vi "50kwh battery decode.vi"(11 "data out":string) -> (0 "F-format string":string[](array[string]), 3 "output array":u32[](array[numeric]))   [LabVIEW 2021]
panel:
  in  "Tab Control":T1(tab)
  out "Main Subsea Battery - 148 V DC, 50 kWh":T2 {"Battery \nPower" scale=0.0..50.0; "SOC" scale=0.0..100.0; "Temp" scale=0.0..50.0; "Bat \nCurrent" scale=0.0..250.0; "Bat\n voltage" scale=0.0..180.0}
  out "Battery Modules":string[][](table)
  out "Battery 1 fault":bool
  out "Battery 2 fault":bool
  out "Battery 3 fault":bool
  out "Battery 4 fault":bool
  out "Battery 5 fault":bool
  out "Battery 1 warn":bool
  out "Battery 2 warn":bool
  out "Battery 3 warn":bool
  out "Battery 4 warn":bool
  out "Battery 5 warn":bool
  out "Battery stat 1":bool
  out "Battery stat 2":bool
  out "Battery stat 3":bool
  out "Battery stat 4":bool
  out "Battery stat 5":bool
  out "Battery Pack 5":T3 {"Power" scale=0.0..10.0; "SOC" scale=0.0..100.0; "Temp" scale=0.0..60.0; "Bat Current" scale=0.0..50.0; "Bat Voltage" scale=0.0..200.0}
  out "Battery Pack 4":T3 {"Power" scale=0.0..10.0; "SOC" scale=0.0..100.0; "Temp" scale=0.0..60.0; "Bat Current" scale=0.0..50.0; "Bat Voltage" scale=0.0..200.0}
  out "Battery Pack 3":T3 {"Power" scale=0.0..10.0; "SOC" scale=0.0..100.0; "Temp" scale=0.0..60.0; "Bat Current" scale=0.0..50.0; "Bat Voltage" scale=0.0..200.0}
  out "Battery Pack 2":T3 {"Power" scale=0.0..10.0; "SOC" scale=0.0..100.0; "Temp" scale=0.0..60.0; "Bat Current" scale=0.0..50.0; "Bat Voltage" scale=0.0..200.0}
  out "Battery Pack 1":T3 {"Power" scale=0.0..10.0; "SOC" scale=0.0..100.0; "Temp" scale=0.0..60.0; "Bat Current" scale=0.0..50.0; "Bat Voltage" scale=0.0..200.0}
  out "length":i32
  out "max .Volt cell":dbl
  out "max. cell ID":dbl
  out "max .C.B.ID":dbl
  out "Min .Volt cell":dbl
  out "Min.Cell.ID":dbl
  out "min.C.B.ID":dbl
  out "x = y?":bool
  out "input":i32
  # "National Institute of Ocean Technology\nMatsya 6000 - Battery System"
  # "kW"
  # "°C"
  # "%"
  # "V"
  # "A"
  # "Bat 4"
  # "Bat 2"
  # "Bat 3"
  # "Bat 1"
  # "Bat 5"
  # "Status"
  # "Warnings"
  # "Faults"
  # "V"
  # "A"
  # "°C"
  # "%"
  # "kW"
  # "V"
  # "A"
  # "°C"
  # "%"
  # "kW"
  # "V"
  # "A"
  # "°C"
  # "%"
  # "kW"
  # "V"
  # "A"
  # "°C"
  # "%"
  # "kW"
  # "V"
  # "A"
  # "°C"
  # "%"
  # "kW"
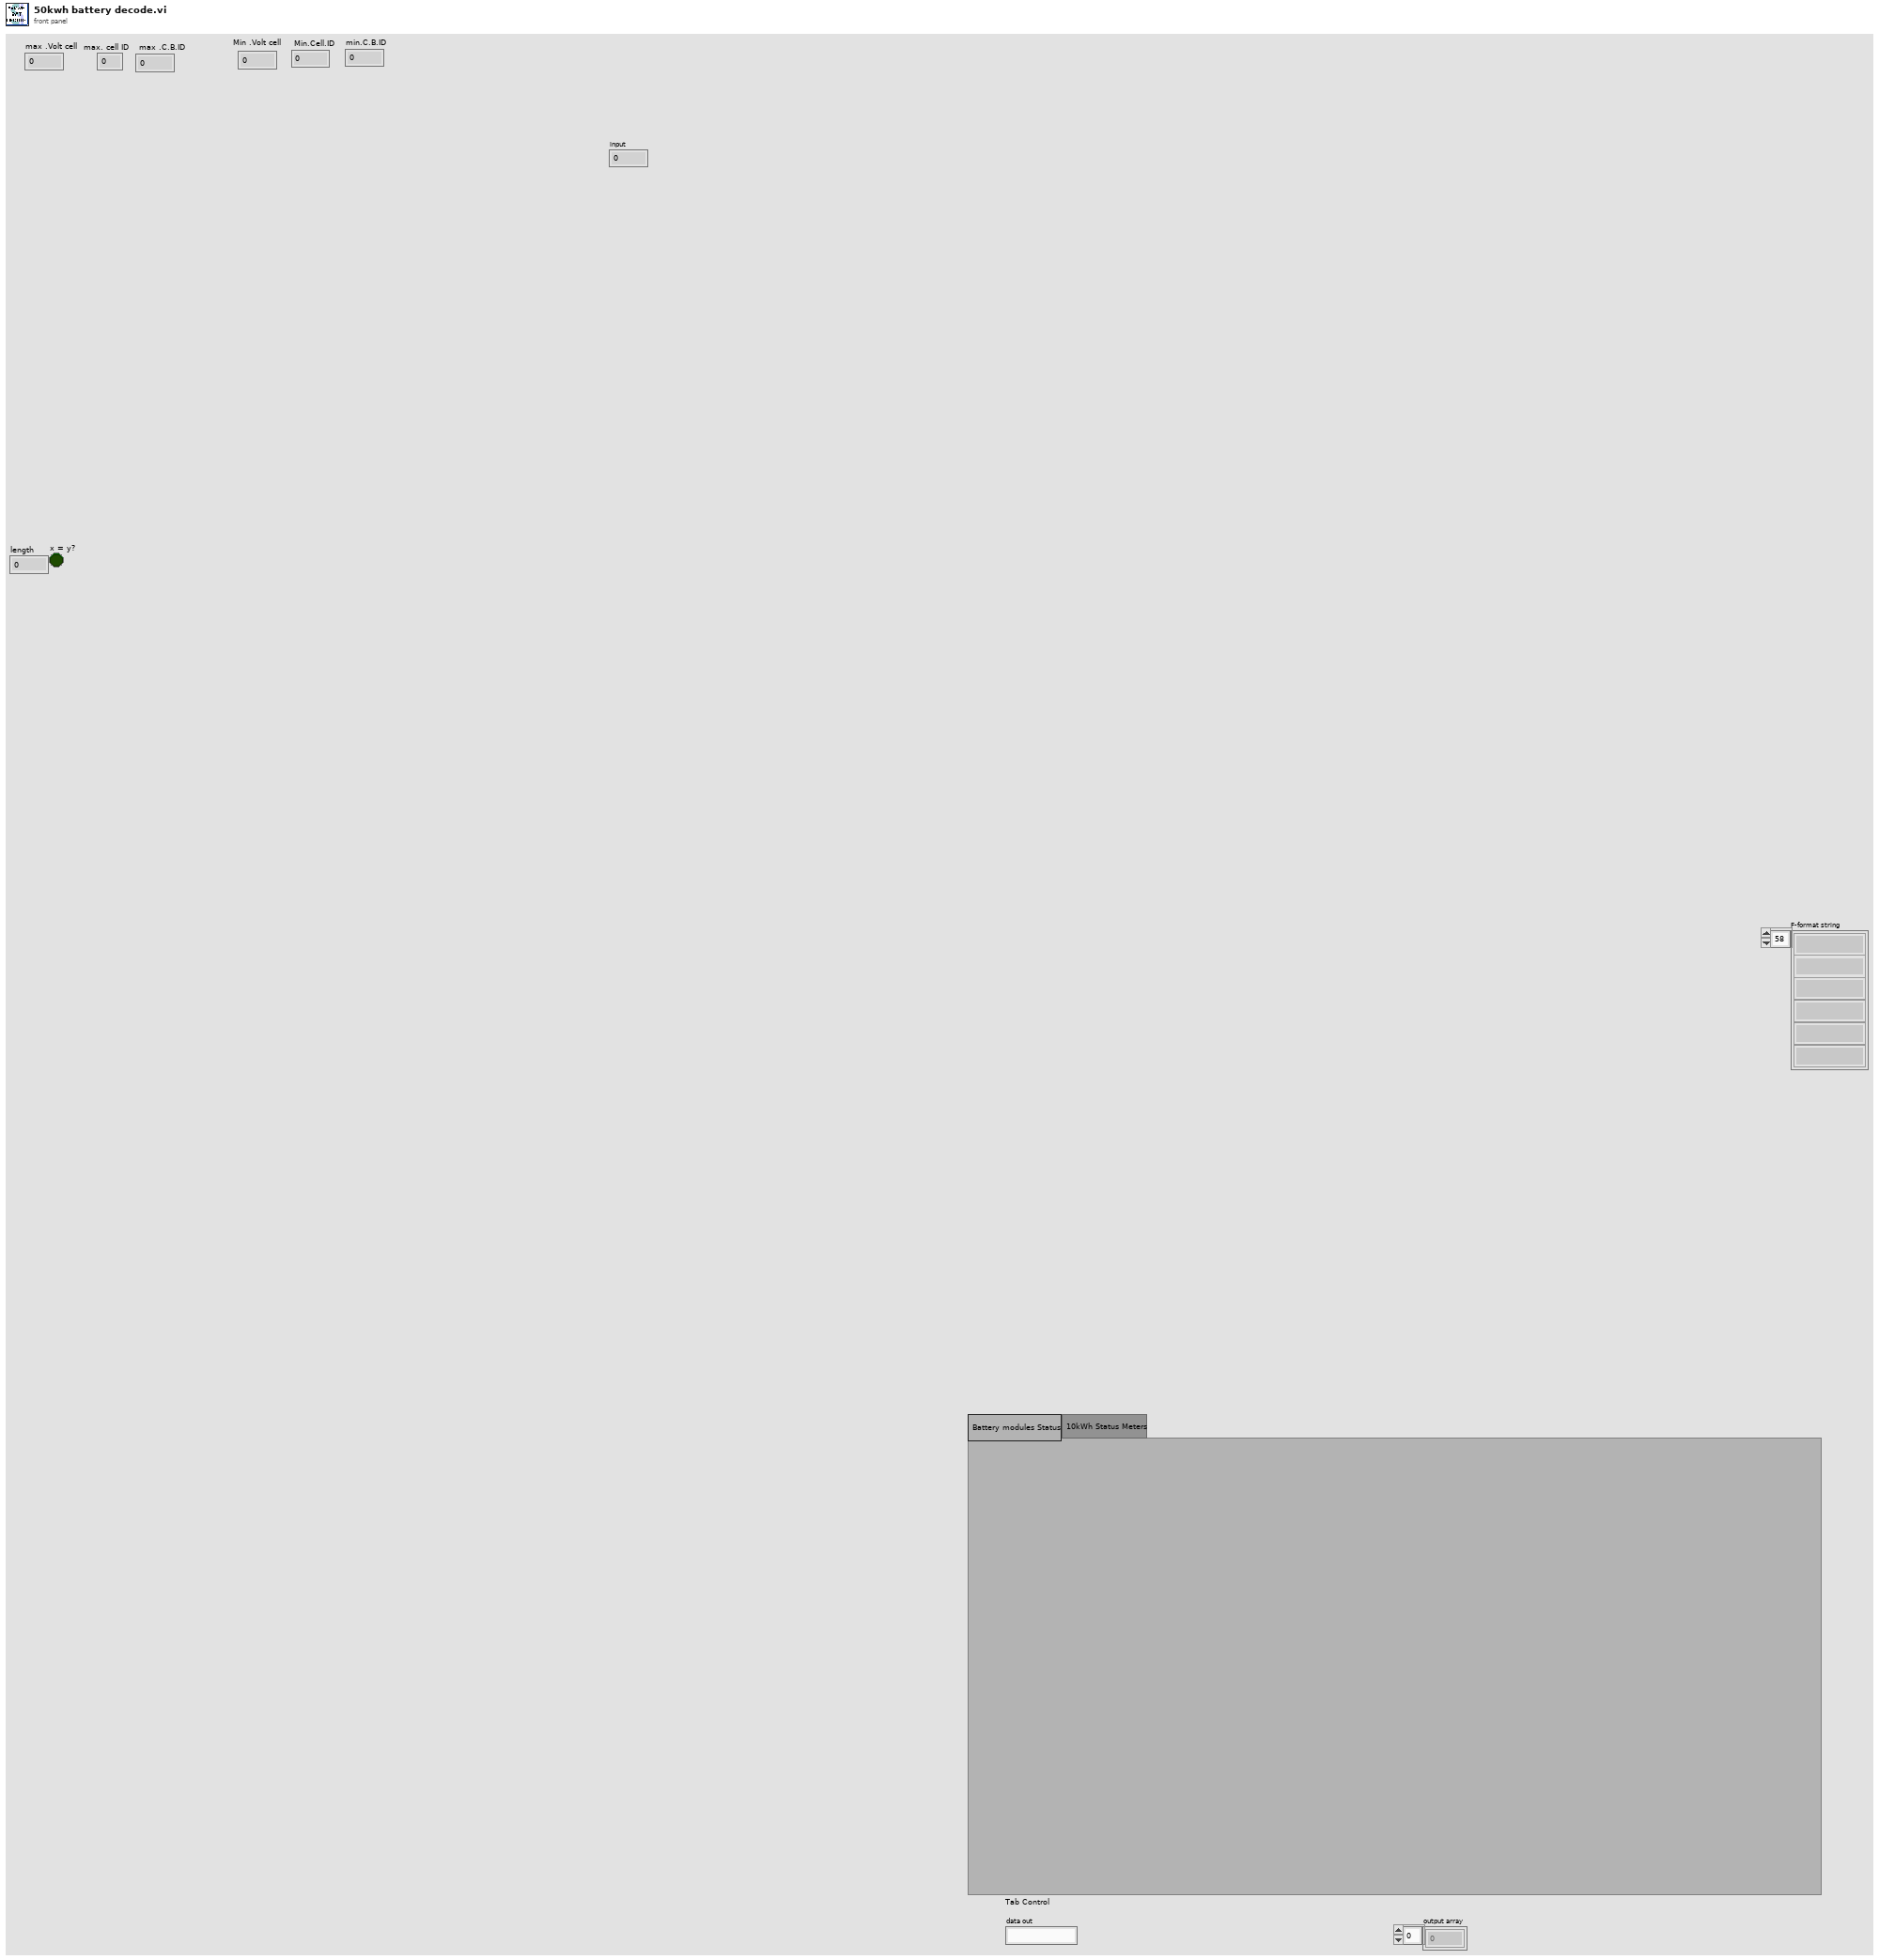
[diagram p1: front panel]
types:
  T1 = enum32{"Battery modules Status", "10kWh Status Meters"}
  T2 = cluster{"Bat\n voltage":u8, "Bat \nCurrent":u8, "Temp":u8, "SOC":u8, "Battery \nPower":sgl}
  T3 = cluster{"Bat Voltage":u16, "Bat Current":u16, "Temp":u8, "SOC":u8, "Power":sgl}
  T4 = cluster{"Numeric":u8, "Numeric":u8, "Numeric":u8, "Numeric":u8, dbl}
  T5 = cluster{u16, u16, "Numeric":u8, "Numeric":u8, dbl}
  T6 = cluster{"Numeric":u8, "Numeric":u8, "Numeric":u8, "Numeric":u8, sgl}
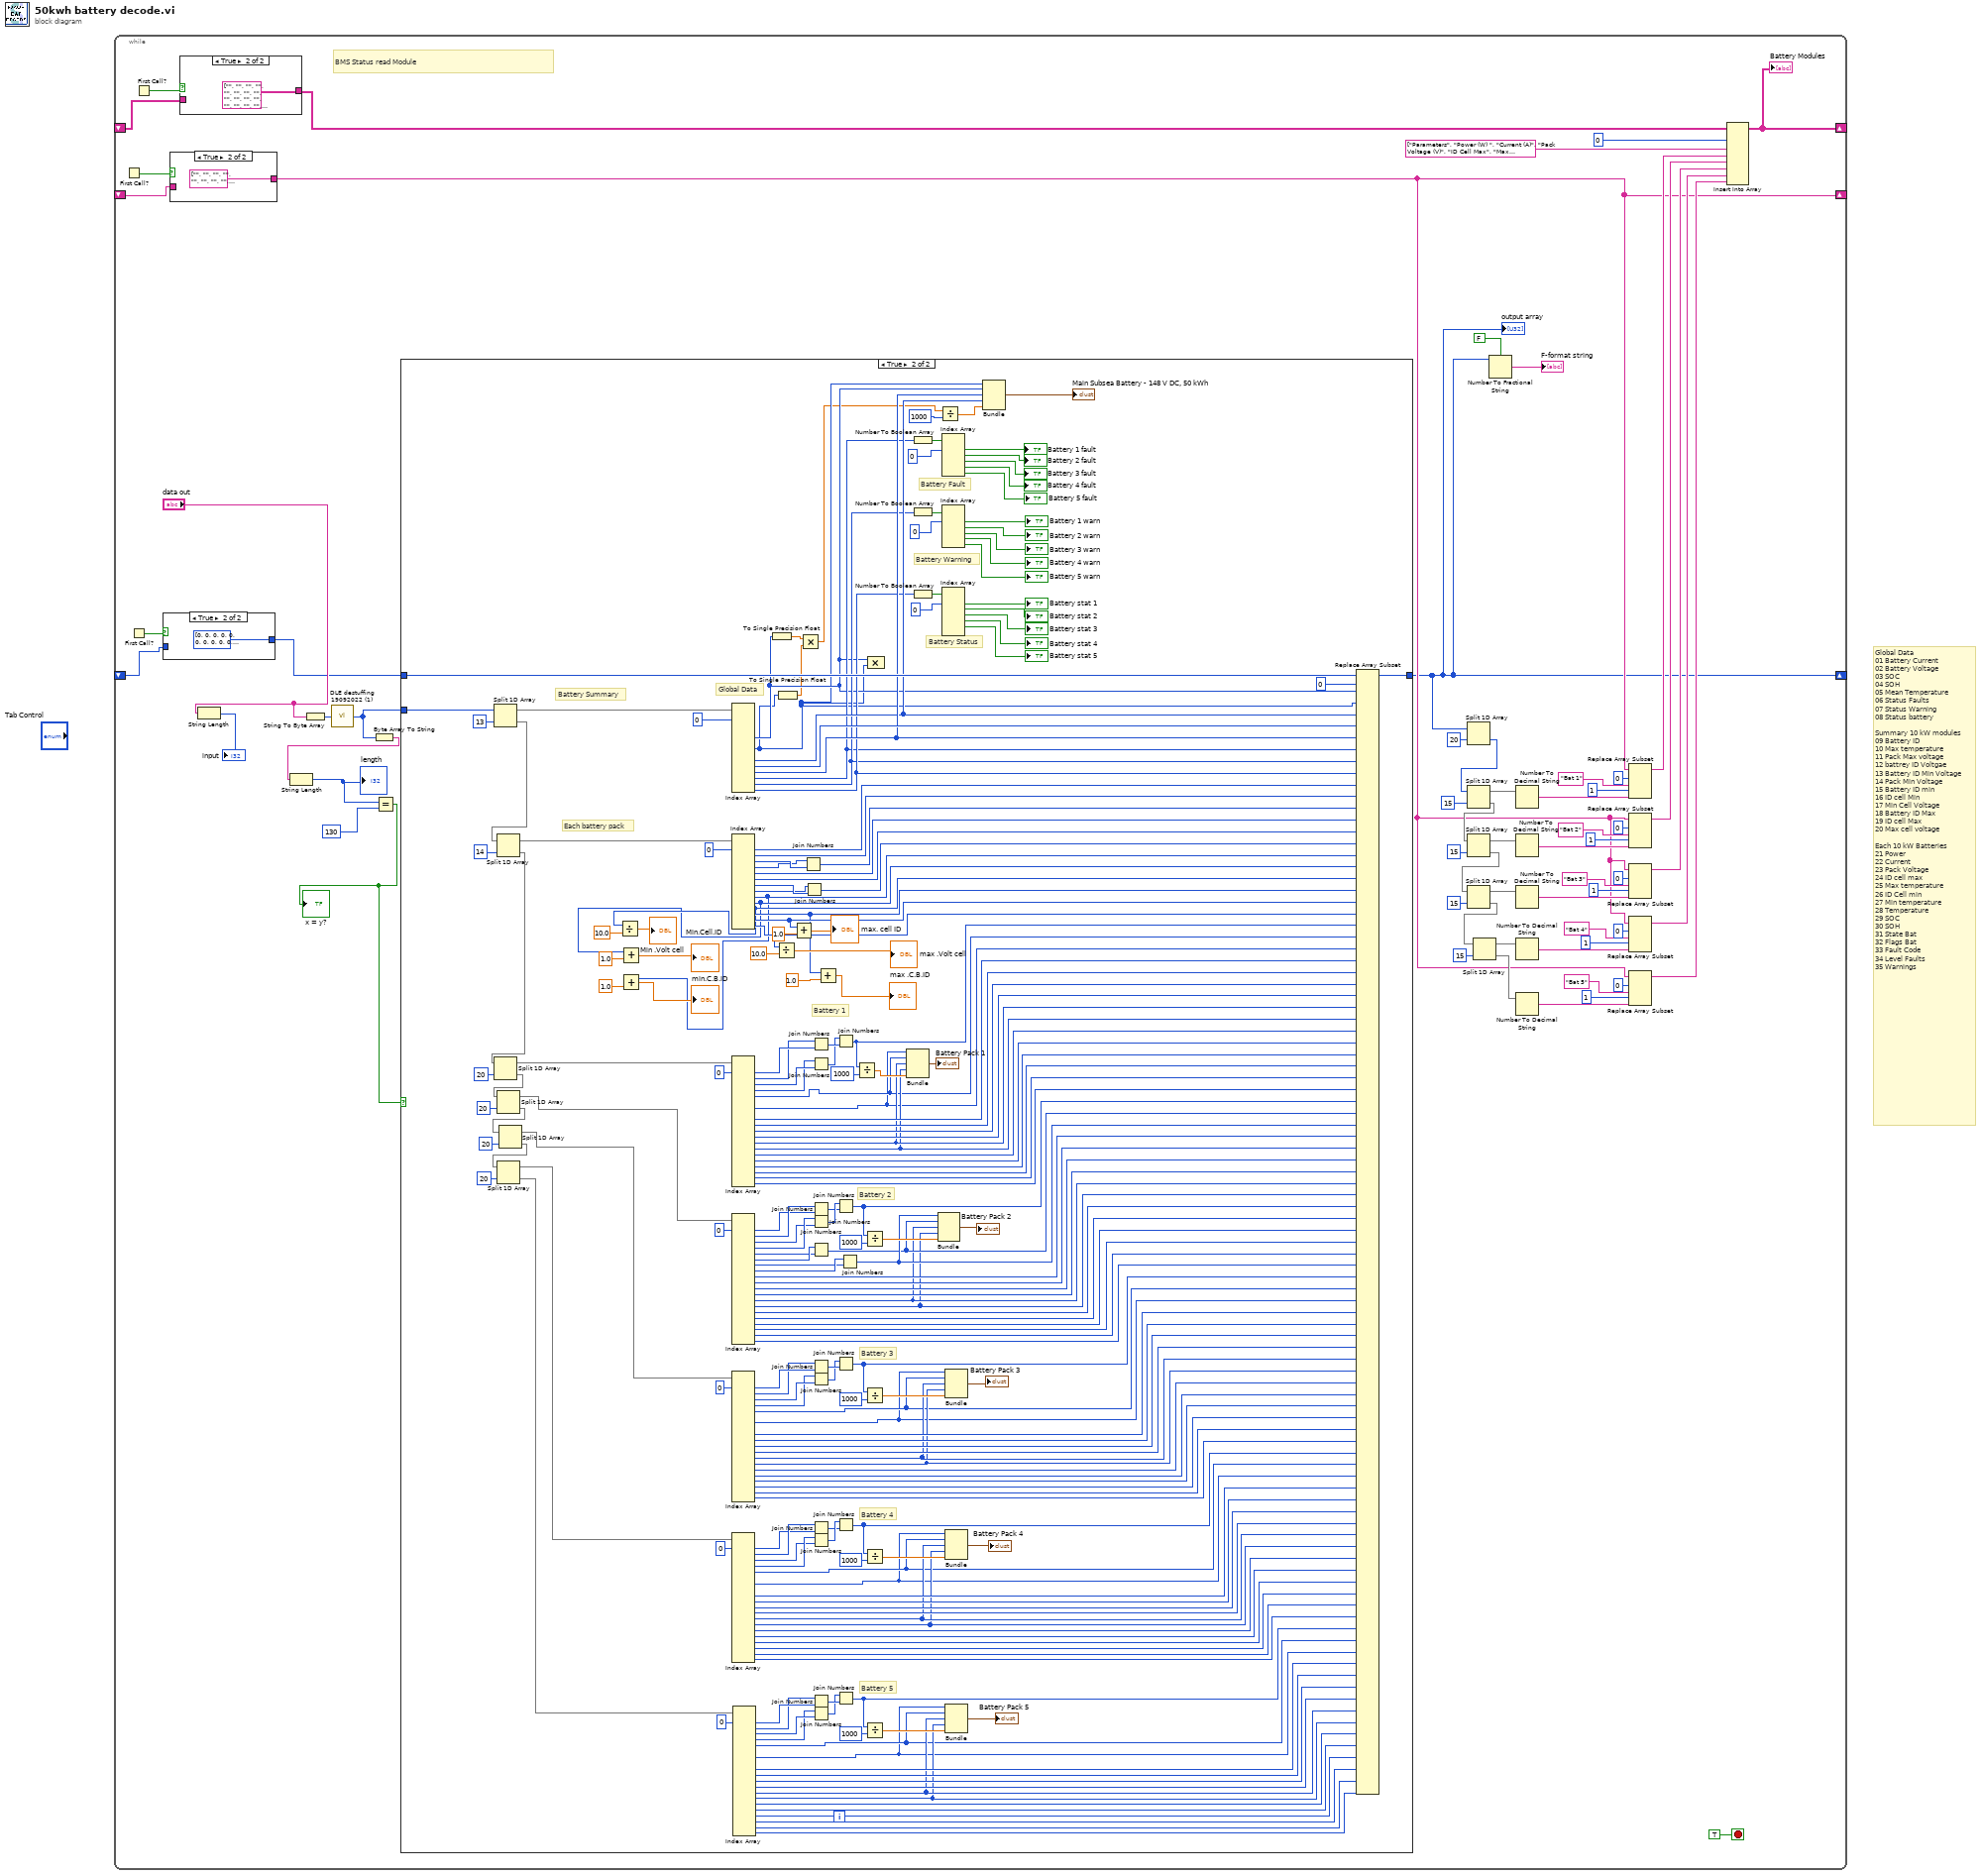
[diagram p0: block diagram]
diagram:
  # "Global Data\n01 Battery Current\n02 Battery Voltage\n03 SOC\n04 SOH\n05 Mean Temperature\n06 Status Faults\n07 Status Warning\n08 Status battery\n\nSummary 10 kW modules\n09 Battery ID\n10 Max temperature\n11 Pack Max voltage\n12 battrey ID Voltgae\n13 Battery ID Min Voltage\n14 Pack Min Voltage\n15 Battery ID min\n16 ID cell Min\n17 Min Cell Voltage\n18 Battery ID Max\n19 ID cell Max\n20 Max cell voltage\n\nEach 10 kW Batteries\n21 Power\n22 Current\n23 Pack Voltage\n24 ID cell max\n25 Max temperature\n26 ID Cell min\n27 Min temperature\n28 Temperature\n29 SOC\n30 SOH\n31 State Bat\n32 Flags Bat\n33 Fault Code\n34 Level Faults\n35 Warnings"
  n1 = while {
    shift-right: [w3] -> _
    shift-left: _ -> [w5]
    shift-right: [w12] -> _
    shift-left: _ -> [w11]
    shift-right: [w8] -> _
    shift-left: _ -> [w7]
    stop <- TRUE stop-if-true
    # "BMS Status read Module"
    n2 = First Call?() -> (First Call?: T/F=w13:bool)
    n3 = First Call?() -> (First Call?: T/F=w6:bool)
    n4 = First Call?() -> (First Call?: T/F=w10:bool)
    n5 = case shown="True" w6 {
      tunnel: [w64 u32[] [0, 0, 0, 0, 0, 0, 0, 0, 0, 0, 0, 0, 0, 0, 0, 0, 0, 0, 0, 0, 0, 0, 0, 0, 0, 0, 0, 0, 0, 0, 0, 0, 0, 0, 0, 0, 0, 0, 0, 0, 0, 0, 0, 0, 0, 0, 0, 0, 0, 0, 0, 0, 0, 0, 0, 0, 0, 0, 0, 0, 0, 0, 0, 0, 0, 0, 0, 0, 0, 0, 0, 0, 0, 0, 0, 0, 0, 0, 0, 0, 0, 0, 0, 0, 0, 0, 0, 0, 0, 0, 0, 0, 0, 0, 0, 0, 0, 0, 0, 0] ("output array")] -> w4
      tunnel: w5 -> [w64 _]
      frame False {
      }
      frame True {
      }
    }
    n6 = case shown="True" w13 {
      tunnel: [w68 string[] ["", "", "", "", "", "", "", "", "", "", "", "", "", "", "", ""] ("decimal integer string")] -> w12
      tunnel: w11 -> [w68 _]
      frame False {
      }
      frame True {
      }
    }
    n7 = case shown="True" w10 {
      tunnel: [w66 string[][] [["", "", "", "", "", "", ""], ["", "", "", "", "", "", ""], ["", "", "", "", "", "", ""], ["", "", "", "", "", "", ""], ["", "", "", "", "", "", ""], ["", "", "", "", "", "", ""], ["", "", "", "", "", "", " "], ["", "", "", "", "", "", ""], ["", "", "", "", "", "", ""], ["", "", "", "", "", "", ""], ["", "", "", "", "", "", ""], ["", "", "", "", "", "", ""], ["", "", "", "", "", "", ""], ["", "", "", "", "", "", ""], ["", "", "", "", "", "", ""], ["", "", "", "", "", "", ""]]] -> w9
      tunnel: w7 -> [w66 _]
      frame False {
      }
      frame True {
      }
    }
    n8 = String Length(string="data out") -> (length=→"input":i32)
    n9 = String To Byte Array(string="data out") -> (unsigned byte array=w19:u8[])
    n10 = call "DLE destuffing 19092022 (1).vi"("DLE stuffed input"=w19) -> ("DLE destuffed output"=w18:u8[])  [unwired: 4 in]
    n11 = Byte Array To String(unsigned byte array=w18) -> (string=w17:string)
    n12 = String Length(string=w17) -> (length=w21:i32)
    "length" <- w21
    n13 = Equal?(x=w21, y=130) -> (x = y?=w15:bool)
    "x = y?" <- w15
    n14 = case shown="True" w15 {
      tunnel: w4 -> [w70 w277]
      tunnel: [w70 w103] -> w3
      tunnel: w18 -> [_ w102]
      frame False {
      }
      frame True {
        # "Battery Fault"
        # "Battery Warning"
        # "Battery Status"
        # "Battery 5"
        # "Battery 4"
        # "Battery 3"
        # "Battery 2"
        # "Battery 1"
        # "Each battery pack"
        # "Battery Summary"
        # "Global Data"
        n15 = Split 1D Array(array=w102, index=13) -> (first subarray=w276:u8[], second subarray=w116:u8[])
        n16 = Split 1D Array(array=w116, index=14) -> (first subarray=w273:u8[], second subarray=w117:u8[])
        n17 = Split 1D Array(array=w117, index=20) -> (first subarray=w234:u8[], second subarray=w283:u8[])
        n18 = Split 1D Array(array=w283, index=20) -> (first subarray=w219:u8[], second subarray=w258:u8[])
        n19 = Split 1D Array(array=w258, index=20) -> (first subarray=w195:u8[], second subarray=w281:u8[])
        n20 = Split 1D Array(array=w281, index=20) -> (first subarray=w164:u8[], second subarray=w165:u8[])
        n21 = Index Array(array=w276, index #1=0 ("index")) -> (element #4=w100:u8, element #6=w98:u8, element #8=w260:u8, element #9=w274:u8, element #10=w261:u8, element #11=w123:u8, element #12=w131:u8, element #13=w134:u8)  [unwired: 12 in, 5 out]
        n22 = Index Array(array=w273, index #1=0 ("index")) -> (element #1=w271:u8, element #2=w270:u8, element #3=w269:u8, element #4=w268:u8, element #5=w266:u8, element #6=w265:u8, element #7=w264:u8, element #8=w263:u8, element #9=w71:u8, element #10=w72:u8, element #11=w75:u8, element #12=w80:u8, element #13=w84:u8, element #14=w87:u8)  [unwired: 13 in]
        n23 = Divide(x=w75, y=10.0) -> (x/y=→"Min .Volt cell":dbl)
        n24 = Add(x=w72, y=1.0) -> (x+y=→"Min.Cell.ID":dbl)
        n25 = Add(x=w71, y=1.0) -> (x+y=→"min.C.B.ID":dbl)
        n26 = Index Array(array=w234, index #1=0 ("index")) -> (element #1=w256:u8, element #2=w255:u8, element #3=w233:u8, element #4=w232:u8, element #5=w101:u8, element #7=w95:u8, element #9=w252:u8, element #10=w251:u8, element #11=w250:u8, element #12=w249:u8, element #13=w236:u8, element #14=w235:u8, element #15=w248:u8, element #16=w247:u8, element #17=w246:u8, element #18=w245:u8, element #19=w244:u8, element #20=w243:u8)  [unwired: 19 in, 2 out]
        n27 = Index Array(array=w219, index #1=0 ("index")) -> (element #1=w221:u8, element #2=w222:u8, element #3=w230:u8, element #4=w231:u8, element #5=w225:u8, element #6=w226:u8, element #7=w227:u8, element #8=w228:u8, element #9=w206:u8, element #10=w205:u8, element #11=w217:u8, element #12=w216:u8, element #13=w115:u8, element #14=w114:u8, element #15=w215:u8, element #16=w214:u8, element #17=w213:u8, element #18=w212:u8, element #19=w211:u8, element #20=w210:u8)  [unwired: 19 in]
        n28 = Index Array(array=w195, index #1=0 ("index")) -> (element #1=w202:u8, element #2=w201:u8, element #3=w197:u8, element #4=w196:u8, element #5=w94:u8, element #7=w93:u8, element #9=w193:u8, element #10=w192:u8, element #11=w191:u8, element #12=w190:u8, element #13=w113:u8, element #14=w112:u8, element #15=w189:u8, element #16=w188:u8, element #17=w187:u8, element #18=w186:u8, element #19=w185:u8, element #20=w184:u8)  [unwired: 19 in, 2 out]
        n29 = Index Array(array=w164, index #1=0 ("index")) -> (element #1=w177:u8, element #2=w178:u8, element #3=w182:u8, element #4=w183:u8, element #5=w92:u8, element #7=w91:u8, element #9=w162:u8, element #10=w161:u8, element #11=w160:u8, element #12=w159:u8, element #13=w111:u8, element #14=w110:u8, element #15=w158:u8, element #16=w157:u8, element #17=w156:u8, element #18=w155:u8, element #19=w154:u8, element #20=w153:u8)  [unwired: 19 in, 2 out]
        n30 = Index Array(array=w165, index #1=0 ("index")) -> (element #1=w172:u8, element #2=w171:u8, element #3=w167:u8, element #4=w166:u8, element #5=w90:u8, element #7=w89:u8, element #9=w151:u8, element #10=w150:u8, element #11=w149:u8, element #12=w148:u8, element #13=w109:u8, element #14=w108:u8, element #15=w147:u8, element #16=w146:u8, element #17=w145:u8, element #18=w144:u8, element #19=w143:u8, element #20=w142:u8)  [unwired: 19 in, 2 out]
        n31 = To Single Precision Float(number=w100) -> (single precision float=w99:sgl)
        n32 = Divide(x=w87, y=10.0) -> (x/y=→"max .Volt cell":dbl)
        n33 = To Single Precision Float(number=w98) -> (single precision float=w97:sgl)
        n34 = Add(x=w84, y=1.0) -> (x+y=→"max. cell ID":dbl)
        n35 = Multiply(x=w99, y=w97) -> (x*y=w96:sgl)
        n36 = Join Numbers(hi=w268, lo=w269) -> ((hi.lo)=w267:u16)
        n37 = Join Numbers(hi=w263, lo=w264) -> ((hi.lo)=w262:u16)
        n38 = Join Numbers(hi=w255, lo=w256) -> ((hi.lo)=w254:u16)
        n39 = Join Numbers(hi=w232, lo=w233) -> ((hi.lo)=w253:u16)
        n40 = Join Numbers(hi=w222, lo=w221) -> ((hi.lo)=w223:u16)
        n41 = Join Numbers(hi=w231, lo=w230) -> ((hi.lo)=w224:u16)
        n42 = Join Numbers(hi=w226, lo=w225) -> ((hi.lo)=w207:u16)
        n43 = Join Numbers(hi=w201, lo=w202) -> ((hi.lo)=w200:u16)
        n44 = Join Numbers(hi=w196, lo=w197) -> ((hi.lo)=w199:u16)
        n45 = Join Numbers(hi=w178, lo=w177) -> ((hi.lo)=w179:u16)
        n46 = Join Numbers(hi=w183, lo=w182) -> ((hi.lo)=w180:u16)
        n47 = Join Numbers(hi=w171, lo=w172) -> ((hi.lo)=w170:u16)
        n48 = Join Numbers(hi=w166, lo=w167) -> ((hi.lo)=w169:u16)
        n49 = Add(x=w80, y=1.0) -> (x+y=→"max .C.B.ID":dbl)
        n50 = Join Numbers(hi=w253, lo=w254) -> ((hi.lo)=w239:u32)
        n51 = Join Numbers(hi=w224, lo=w223) -> ((hi.lo)=w218:u32)
        n52 = Join Numbers(hi=w199, lo=w200) -> ((hi.lo)=w194:u32)
        n53 = Join Numbers(hi=w180, lo=w179) -> ((hi.lo)=w163:u32)
        n54 = Join Numbers(hi=w169, lo=w170) -> ((hi.lo)=w152:u32)
        n55 = Join Numbers(hi=w228, lo=w227) -> ((hi.lo)=w208:u16)
        n56 = Divide(x=w239, y=u16 1000) -> (x/y=w237:dbl)
        n57 = Divide(x=w218, y=u16 1000) -> (x/y=w209:dbl)
        n58 = Divide(x=w194, y=u16 1000) -> (x/y=w204:dbl)
        n59 = Divide(x=w163, y=u16 1000) -> (x/y=w175:dbl)
        n60 = Divide(x=w152, y=u16 1000) -> (x/y=w174:dbl)
        n61 = Compound Arithmetic op=MULTIPLY(w100, w98) -> ()  [unwired: 1 out]
        n62 = Bundle("Numeric"=w95, "Numeric"=w101, "Numeric"=w236, "Numeric"=w235, w237) -> (→"Battery Pack 1":T4)  [unwired: 1 in]
        n63 = Number To Boolean Array(number=w123) -> (Boolean array=w125:bool[])
        n64 = Number To Boolean Array(number=w131) -> (Boolean array=w132:bool[])
        n65 = Number To Boolean Array(number=w134) -> (Boolean array=w141:bool[])
        n66 = Bundle(w208, w207, "Numeric"=w115, "Numeric"=w114, w209) -> (→"Battery Pack 2":T5)  [unwired: 1 in]
        n67 = Divide(x=w96, y=u16 1000) -> (x/y=w241:sgl)
        n68 = Index Array(array=w125, index #1=0 ("index")) -> (element #1=→"Battery 1 fault":bool, element #2=→"Battery 2 fault":bool, element #3=→"Battery 3 fault":bool, element #4=→"Battery 4 fault":bool, element #5=→"Battery 5 fault":bool)  [unwired: 4 in]
        n69 = Index Array(array=w132, index #1=0 ("index")) -> (element #1=→"Battery 1 warn":bool, element #2=→"Battery 2 warn":bool, element #3=→"Battery 3 warn":bool, element #4=→"Battery 4 warn":bool, element #5=→"Battery 5 warn":bool)  [unwired: 4 in]
        n70 = Index Array(array=w141, index #1=0 ("index")) -> (element #1=→"Battery stat 1":bool, element #2=→"Battery stat 2":bool, element #3=→"Battery stat 3":bool, element #4=→"Battery stat 4":bool, element #5=→"Battery stat 5":bool)  [unwired: 5 in, 1 out]
        n71 = Bundle("Numeric"=w93, "Numeric"=w94, "Numeric"=w113, "Numeric"=w112, w204) -> (→"Battery Pack 3":T4)  [unwired: 1 in]
        n72 = Bundle("Numeric"=w91, "Numeric"=w92, "Numeric"=w111, "Numeric"=w110, w175) -> (→"Battery Pack 4":T4)  [unwired: 1 in]
        n73 = Bundle("Numeric"=w89, "Numeric"=w90, "Numeric"=w109, "Numeric"=w108, w174) -> (→"Battery Pack 5":T4)  [unwired: 1 in]
        n74 = Bundle("Numeric"=w98, "Numeric"=w100, "Numeric"=w261, "Numeric"=w260, w241) -> (→"Main Subsea Battery - 148 V DC, 50 kWh":T6)  [unwired: 1 in]
        n75 = Replace Array Subset(array=w277, new element #1=w100, index #1=0 ("index"), new element #2=w98, new element #3=w260, new element #4=w274, new element #5=w261, new element #6=w123, new element #7=w131, new element #8=w134, new element #9=w271, new element #10=w270, new element #11=w267, new element #12=w266, new element #13=w265, new element #14=w262, new element #15=w71, new element #16=w72, new element #17=w75, new element #18=w80, new element #19=w84, new element #20=w87, new element #21=w239, new element #22=w101, new element #23=w95, new element #24=w252, new element #25=w251, new element #26=w250, new element #27=w249, new element #28=w236, new element #29=w235, new element #30=w248, new element #31=w247, new element #32=w246, new element #33=w245, new element #34=w244, new element #35=w243, new element #36=w218, new element #37=w207, new element #38=w208, new element #39=w206, new element #40=w205, new element #41=w217, new element #42=w216, new element #43=w115, new element #44=w114, new element #45=w215, new element #46=w214, new element #47=w213, new element #48=w212, new element #49=w211, new element #50=w210, new element #51=w194, new element #52=w94, new element #53=w93, new element #54=w193, new element #55=w192, new element #56=w191, new element #57=w190, new element #58=w113, new element #59=w112, new element #60=w189, new element #61=w188, new element #62=w187, new element #63=w186, new element #64=w185, new element #65=w184, new element #66=w163, new element #67=w92, new element #68=w91, new element #69=w162, new element #70=w161, new element #71=w160, new element #72=w159, new element #73=w111, new element #74=w110, new element #75=w158, new element #76=w157, new element #77=w156, new element #78=w155, new element #79=w154, new element #80=w153, new element #81=w152, new element #82=w90, new element #83=w89, new element #84=w151, new element #85=w150, new element #86=w149, new element #87=w148, new element #88=w109, new element #89=w108, new element #90=w147, new element #91=w146, new element #92=w145, new element #93=w144, new element #94=w143, new element #95=w142) -> (w103:u32[])  [unwired: 94 in]
      }
    }
    "output array" <- w3
    n76 = Split 1D Array(array=w3, index=20) -> (second subarray=w23:u32[])  [unwired: 1 out]
    n77 = Split 1D Array(array=w23, index=15) -> (first subarray=w32:u32[], second subarray=w34:u32[])
    n78 = Split 1D Array(array=w34, index=15) -> (first subarray=w33:u32[], second subarray=w30:u32[])
    n79 = Split 1D Array(array=w30, index=15) -> (first subarray=w29:u32[], second subarray=w27:u32[])
    n80 = Split 1D Array(array=w27, index=15) -> (first subarray=w25:u32[], second subarray=w24:u32[])
    n81 = Number To Fractional String(use system decimal point (T)=FALSE, number=w3) -> (F-format string=→"F-format string":string[])  [unwired: 2 in]
    n82 = Number To Decimal String(number=w33) -> (decimal integer string=w49:string[])  [unwired: 1 in]
    n83 = Number To Decimal String(number=w32) -> (decimal integer string=w57:string[])  [unwired: 1 in]
    n84 = Number To Decimal String(number=w29) -> (decimal integer string=w40:string[])  [unwired: 1 in]
    n85 = Number To Decimal String(number=w25) -> (decimal integer string=w22:string[])  [unwired: 1 in]
    n86 = Number To Decimal String(number=w24) -> (decimal integer string=w26:string[])  [unwired: 1 in]
    n87 = Replace Array Subset(array=w12, new element #1="Bat 1" ("new element/subarray"), index #1=0 ("index"), new element #2=w57, index #2=1 ("index")) -> (w53:string[])
    n88 = Replace Array Subset(array=w12, new element #1="Bat 2" ("new element/subarray"), index #1=0 ("index"), new element #2=w49, index #2=1 ("index")) -> (w48:string[])
    n89 = Replace Array Subset(array=w12, new element #1="Bat 3" ("new element/subarray"), index #1=0 ("index"), new element #2=w40, index #2=1 ("index")) -> (w47:string[])
    n90 = Replace Array Subset(array=w12, new element #1="Bat 4" ("new element/subarray"), index #1=0 ("index"), new element #2=w22, index #2=1 ("index")) -> (w39:string[])
    n91 = Replace Array Subset(array=w12, new element #1="Bat 5" ("new element/subarray"), index #1=0 ("index"), new element #2=w26, index #2=1 ("index")) -> (w38:string[])
    n92 = Insert Into Array(array=w9, index (col)=0 ("index (row)"), new element #1=string[] ["Parameters", "Power (W) ", "Current (A)", "Pack Voltage (V)", "ID Cell Max", "Max Temperature(°C)", "ID Cell min", "Min Temeperature (°C)", "Temperature (°C)", "SOC (%)", "SOH (%)", "State battery", "Flags", "Faults", "Level", "Warnings"] ("Table Control"), new element #2=w53, new element #3=w48, new element #4=w47, new element #5=w39, new element #6=w38) -> (w8:string[][])  [unwired: 1 in]
    "Battery Modules" <- w8
  }
